vi "ClickOnPieceOperations.vi"(9 "Input DataBase":T1, 10 "Off Board?":bool, 11 "Clicked Position":i32[](array[numeric])) -> (2 "Output DataBase":T1, 3 "Output State":T8)   [LabVIEW 2019]
uses:
  #typedef_DataBase.ctl
  #typedef_SquareType.ctl
  #typedef_Color.ctl
  #typedef_Piece.ctl
  #typedef_PieceType.ctl
  #typedef_SquareLook.ctl
  #typedef_SpecialMoves.ctl
  #typedef_ProgramStates.ctl
panel:
  out "?":u16[][](array[ring])
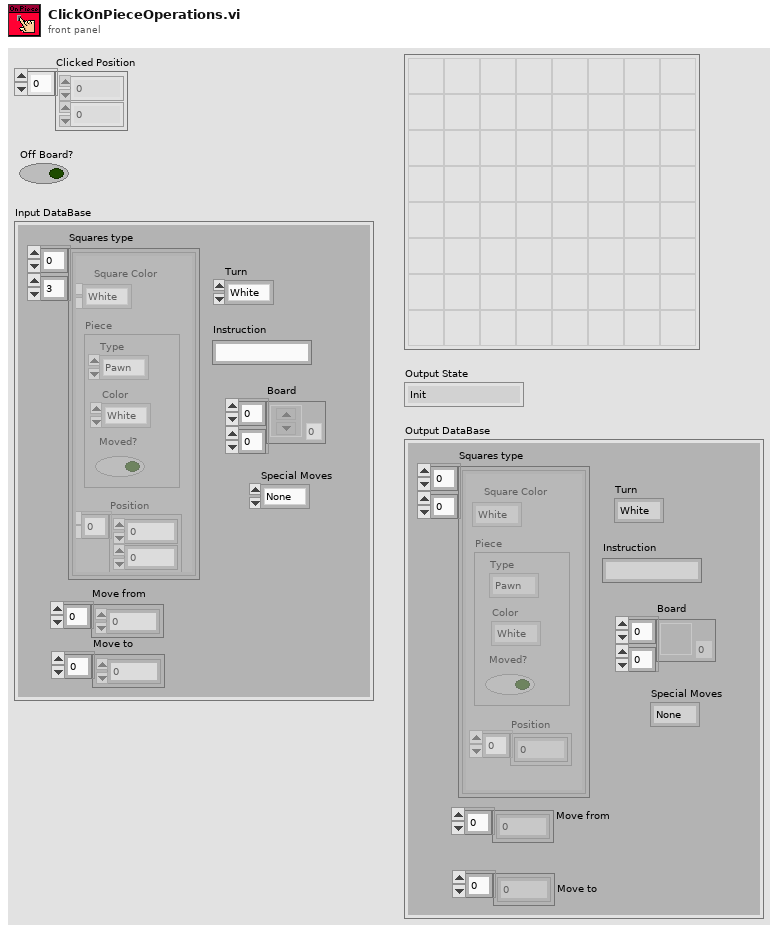
[diagram p1: front panel]
types:
  T1 = typedef "#typedef_DataBase.ctl" = cluster{"Squares type":T2[][], "Turn":T3, "Move from":i32[], "Move to":i32[], "Instruction":string, "Board":T6[][], "Special Moves":T7}
  T2 = typedef "#typedef_SquareType.ctl" = cluster{"Square Color":T3, "Position":i32[], "Piece":T4}
  T3 = typedef "#typedef_Color.ctl" = enum16{"White", "Black"}
  T4 = typedef "#typedef_Piece.ctl" = cluster{"Type":T5, "Color":T3, "Moved?":bool}
  T5 = typedef "#typedef_PieceType.ctl" = enum16{"None", "Pawn", "Knight", "Bishop", "Rook", "Queen", "King"}
  T6 = typedef "#typedef_SquareLook.ctl" = u16
  T7 = typedef "#typedef_SpecialMoves.ctl" = enum16{"None", "Last Square", "Beat in the Passage", "Short Castle", "Long Castle"}
  T8 = typedef "#typedef_ProgramStates.ctl" = enum16{"Init", "Clicking on Piece", "Clicking on Square", "Checking Movement", "Checking King  ", "Checking if Mate", "End"}
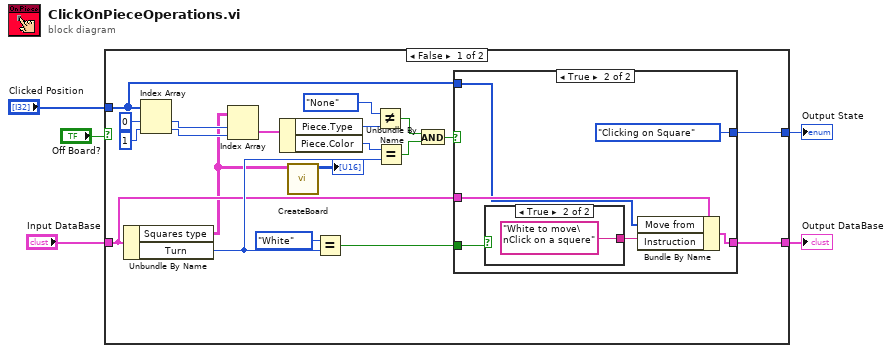
[diagram p0: block diagram]
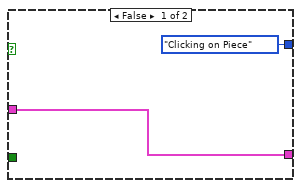
[diagram p2: hidden frame]
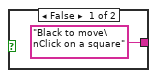
[diagram p3: hidden frame]
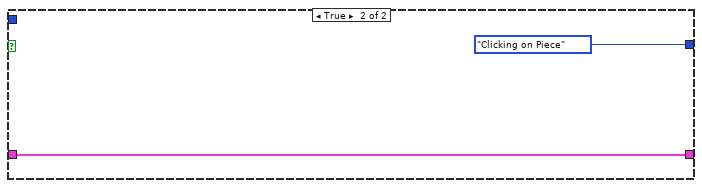
[diagram p4: hidden frame]
diagram:
  n1 = case shown="False" "Off Board?" {
    tunnel: "Input DataBase" -> [w10 w37]
    tunnel: [w9 w37] -> w5
    tunnel: [w11 #typedef_ProgramStates."Clicking on Piece" ("Conditional State")] -> w4
    tunnel: "Clicked Position" -> [w6 _]
    frame False {
      n2 = Unbundle By Name(w10) -> ("Squares type"=w8:T2[][], "Turn"=w14:T3)
      n3 = Index Array(array=w6, index #1=0 ("index"), index #2=1 ("index")) -> (element #1=w23:i32, element #2=w22:i32)
      n4 = Index Array(array=w8, index (row)=w23, index (col)=w22) -> (element=w21:T2)
      n5 = Unbundle By Name(w21) -> ("Piece.Type"=w20:T5, "Piece.Color"=w18:T3)
      n6 = call "CreateBoard.vi"("Squares type"=w8) -> ("Board"=→"?":u16[][])  [unwired: 10 in]
      n7 = Equal?(x=#typedef_Color."White", y=w14) -> (x = y?=w12:bool)
      n8 = Not Equal?(x=#typedef_PieceType."None", y=w20) -> (x != y?=w16:bool)
      n9 = Equal?(x=w18, y=w14) -> (x = y?=w17:bool)
      n10 = And(x=w16, y=w17) -> (x .and. y?=w15:bool)
      n11 = case shown="True" w15 {
        tunnel: w12 -> [_ w33]
        tunnel: [#typedef_ProgramStates."Clicking on Piece" ("Conditional State") #typedef_ProgramStates."Clicking on Square" ("Conditional State")] -> w11
        tunnel: w10 -> [w26 w32]
        tunnel: [w26 w30] -> w9
        tunnel: w6 -> [_ w28]
        frame False {
        }
        frame True {
          n12 = case shown="True" w33 {
            tunnel: ["Black to move\nClick on a square" "White to move\nClick on a squere"] -> w31
            frame False {
            }
            frame True {
            }
          }
          n13 = Bundle By Name(cluster=w32, "Move from"=w28, "Instruction"=w31) -> (w30:T1)
        }
      }
    }
    frame True {
    }
  }
  "Output State" <- w4
  "Output DataBase" <- w5
